vi "Measurement UI.vi"() -> ()   [LabVIEW 2021, in "channelGanging.lvlib"]
uses:
  channelGanging.lvlib
panel:
  in  "MeasGraphs":T1(tab)
  out "SourceCurrentGraph":waveform(dbl)[](graph) caption="AC"
  out "SourceVoltageGraph":waveform(dbl)[](graph) caption="AC"
  out "LoadCurrentGraph":waveform(dbl)[](graph) caption="AC"
  out "LoadVoltageGraph":waveform(dbl)[](graph) caption="AC"
  in  "Load channel mode":enum32{"Master", "Slave", "Slave- inverted"}[](array[ring])
  in  "Load resource names":string[](array[string])
  in  "Load input channels":i32[](array[numeric])
  in  "Source channel mode":enum32{"Master", "Slave", "Slave- inverted"}[](array[ring])
  in  "Source resource names":string[](array[string])
  in  "Source input channels":i32[](array[numeric])
  out "Load currents":dbl[](array[numeric])
  out "Load voltages":dbl[](array[numeric])
  out "Source currents":dbl[](array[numeric])
  out "Source voltages":dbl[](array[numeric])
  out "dt":dbl[](array[numeric])
  in  "MeasConfigurations":enum32{"Source Config", "Load Config"}(tab)
  in  "Source transient response":enum32{"Fast", "Normal", "Slow"}(ring) caption="TRANSIENT RESPONSE"
  in  "Source voltage level range":dbl=20.0 caption="VOLTAGE LEVEL RANGE" format="%#_6pV"
  in  "Source voltage level":dbl=2.0 caption="VOLTAGE LEVEL" format="%#_6pV"
  in  "Source channel parameters":T2(array[cluster]) caption="CHANNEL PARAMETERS"
  in  "Source current limit high":dbl=50.0 caption="CURRENT LIMIT HIGH" format="%#_6pA"
  in  "Source current limit range":dbl=40.0 caption="CURRENT LIMIT RANGE" format="%#_6pA"
  in  "Source limit symmetry":enum32{"Asymmetric", "Symmetric"}(ring) caption="LIMIT SYMMETRY"
  in  "Source current limit low":dbl=-0.6 caption="CURRENT  LIMIT LOW" format="%#_6pA"
  in  "Source system configuration":enum32{"Parallel", "Series"}(ring) caption="SYSTEM CONFIG"
  in  "Source sense":enum32{"Remote", "Local"}(ring) caption="SENSE"
  in  "Source aperture time":dbl=0.01 caption="APERTURE TIME" format="%.3ps"
  in  "Source compliance":string="Compliance"
  in  "Source timing":string="Timings"
  in  "Measurement time":dbl=1.0 caption="MEASUREMENT TIME" format="%.3ps"
  in  "Load transient response":enum32{"Fast", "Normal", "Slow"}(ring)=enum."Normal" caption="TRANSIENT RESPONSE"
  in  "Load timing":string="Timings"
  in  "Load compliance":string="Compliance"
  in  "Load aperture time":dbl=0.01 caption="APERTURE TIME" format="%.3ps"
  in  "Load Sense":enum32{"Remote", "Local"}(ring) caption="SENSE"
  in  "Load system configuration":enum32{"Parallel", "Series"}(ring) caption="SYSTEM CONFIG"
  in  "Load voltage limit low":dbl caption="VOLTAGE  LIMIT LOW" format="%#_6pV"
  in  "Load limit symmetry":enum32{"Asymmetric", "Symmetric"}(ring) caption="LIMIT SYMMETRY"
  in  "Load voltage limit range":dbl=6.0 caption="VOLTAGE LIMIT RANGE" format="%#_6pV"
  in  "Load voltage limit high":dbl=inf caption="VOLTAGE LIMIT HIGH" format="%#_6p"
  in  "Load current Level":dbl=30.0 caption="CURRENT LEVEL" format="%#_6pA"
  in  "Load current level range":dbl=50.0 caption="CURRENT LEVEL RANGE" format="%#_6pA"
  in  "Load channel parameters":T3(array[cluster]) caption="CHANNEL PARAMETERS"
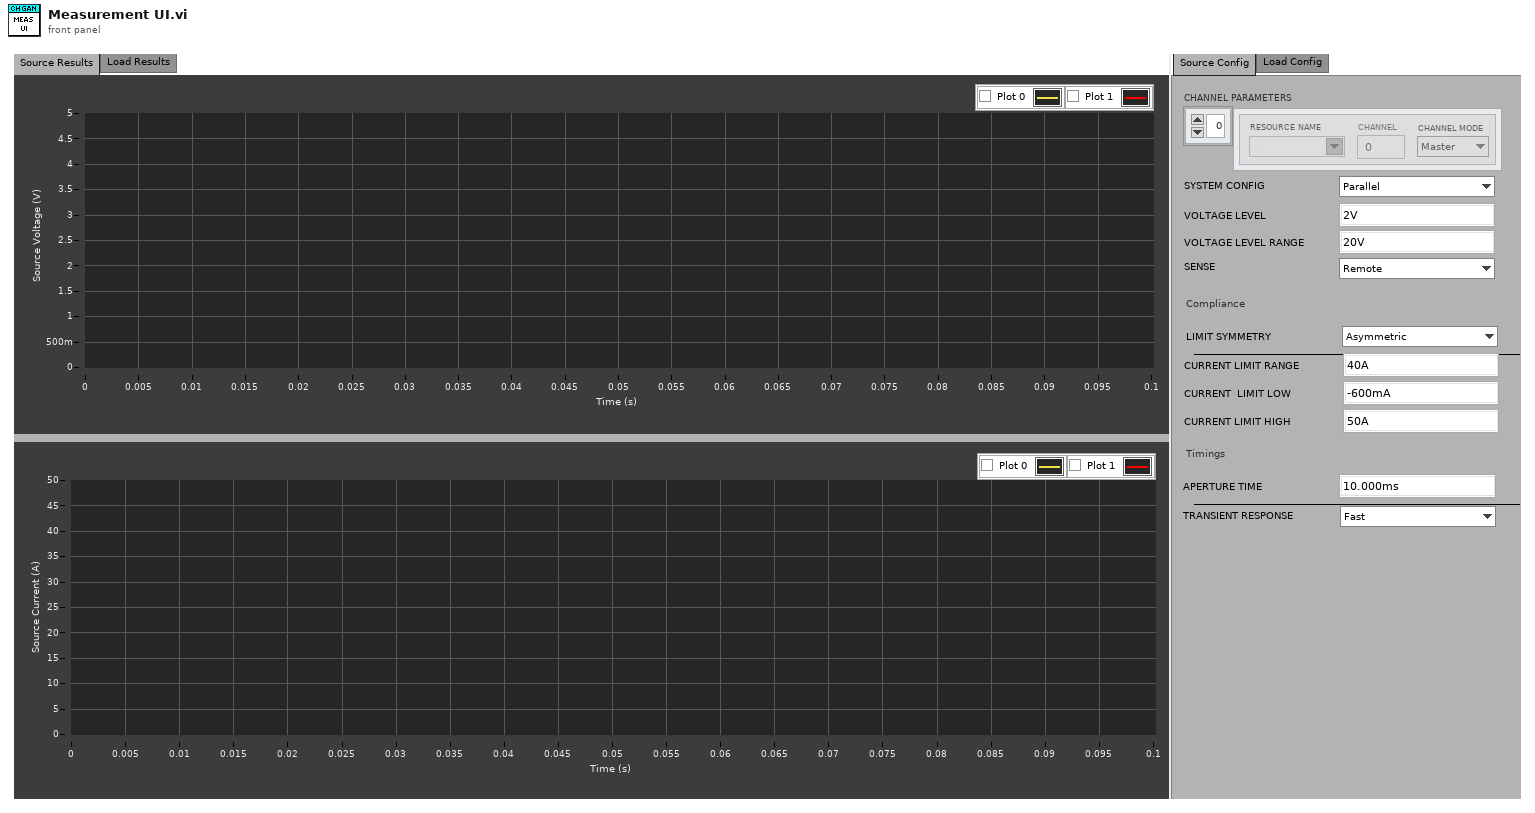
[diagram p1: front panel]
types:
  T1 = enum32{"Source Results", "Load Results", "Hidden Controls"}
  T2 = cluster{"PPSChannelMode":enum32{"Master", "Slave", "Slave- inverted"}, "PPSResourceName":refnum<k15>, "Input channel":i32}[]
  T3 = cluster{"EloadChannelMode":enum32{"Master", "Slave", "Slave- inverted"}, "EloadResourceName":refnum<k15>, "Load channel":i32}[]
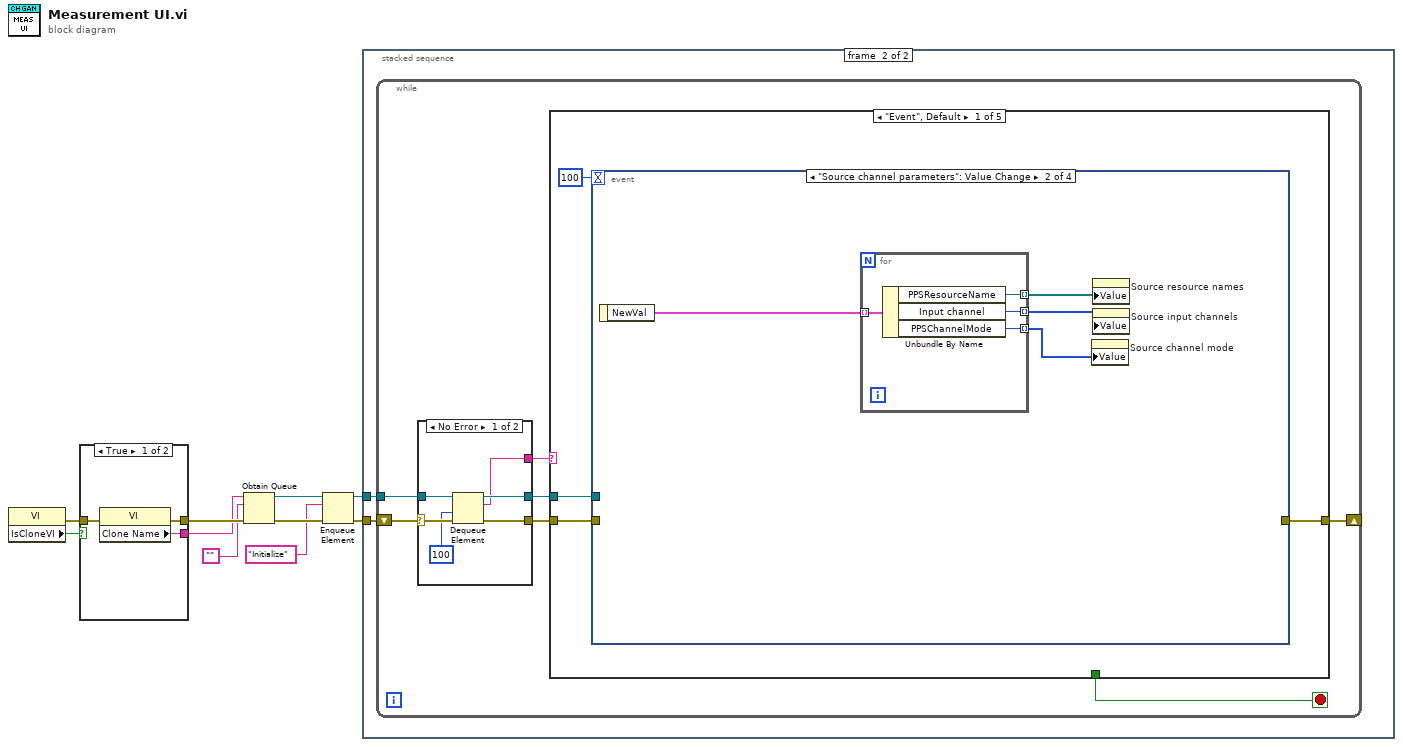
[diagram p0: block diagram]
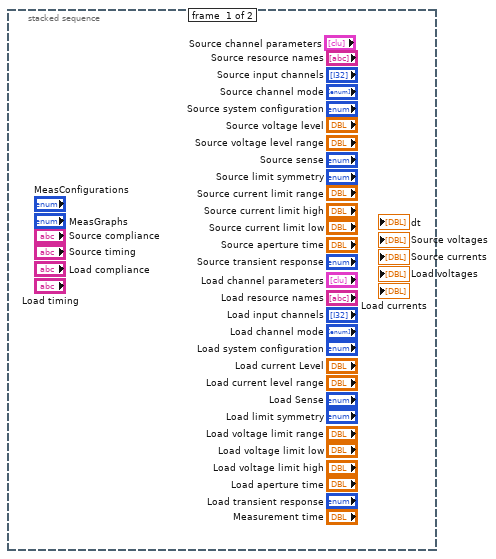
[diagram p2: hidden frame]
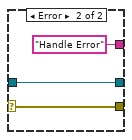
[diagram p3: hidden frame]
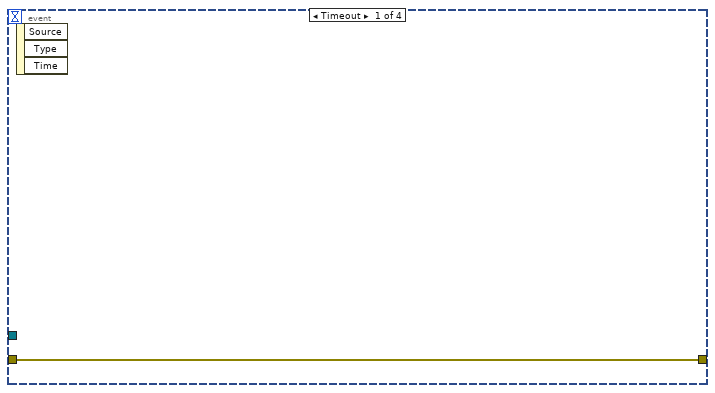
[diagram p4: hidden frame]
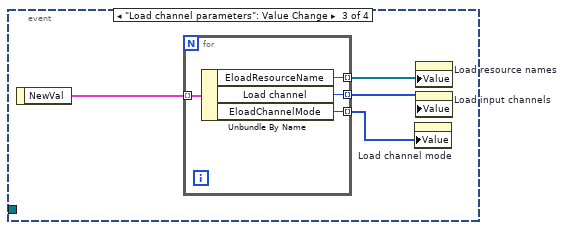
[diagram p5: hidden frame]
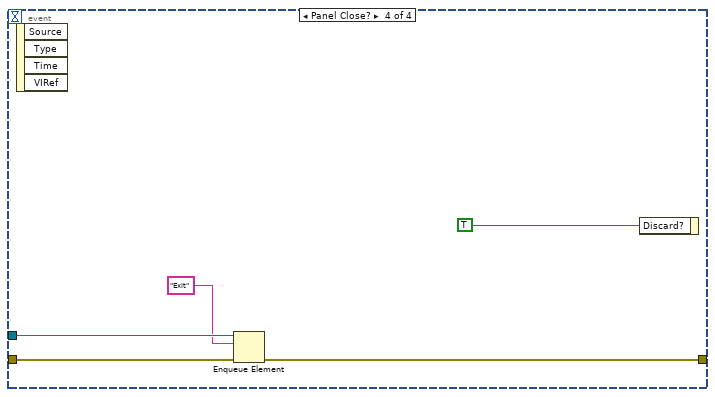
[diagram p6: hidden frame]
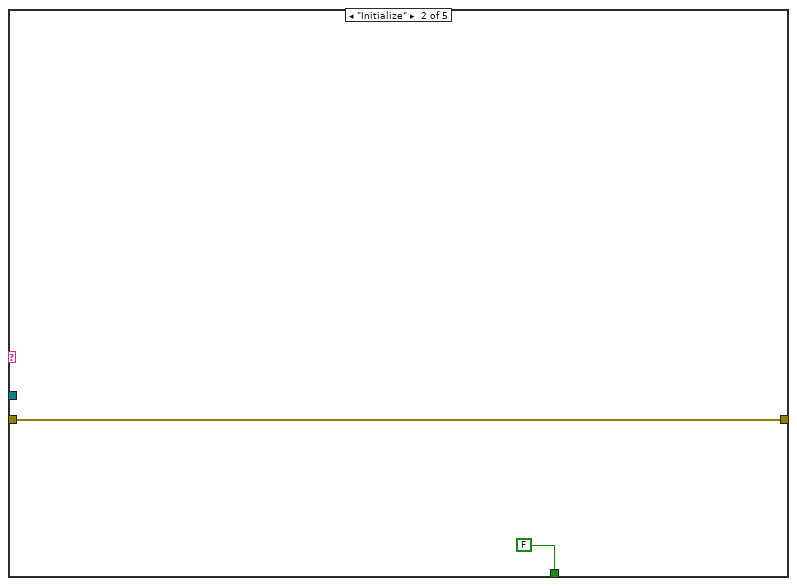
[diagram p7: hidden frame]
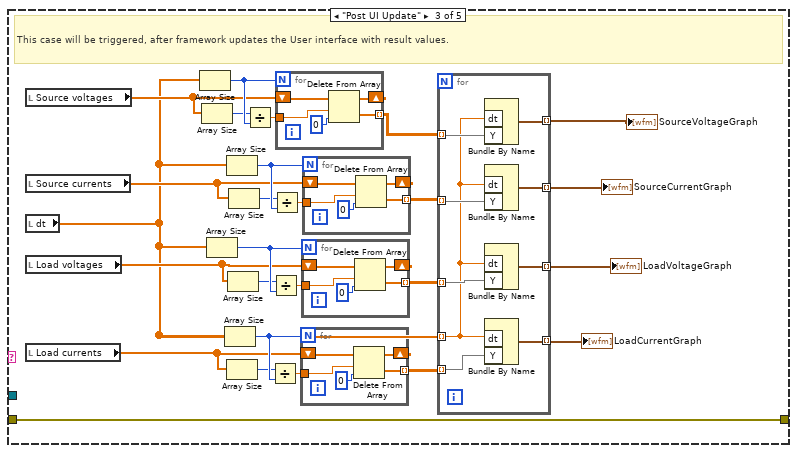
[diagram p8: hidden frame]
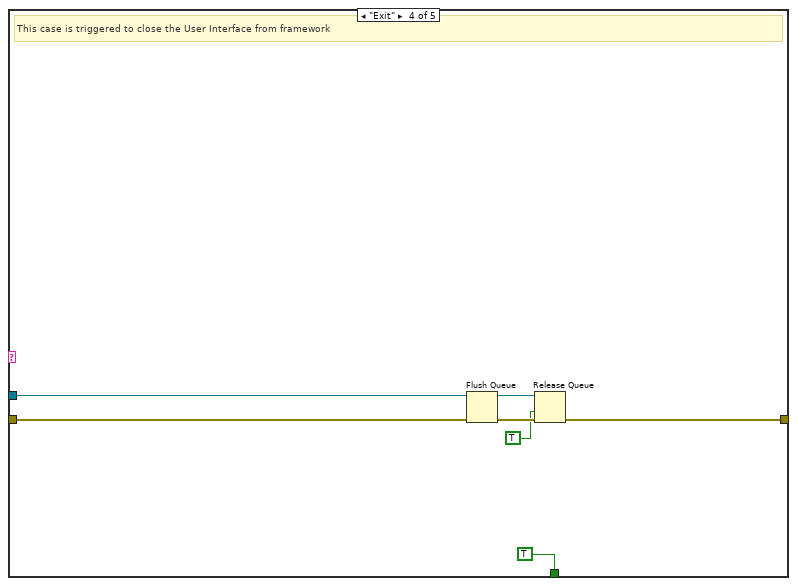
[diagram p9: hidden frame]
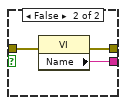
[diagram p11: hidden frame]
diagram:
  n1 = property class="VI"() -> (error out=w1:errorcluster, "IsCloneVI"=w2:bool)  [unwired: 2 in, 1 out]
  n2 = case shown="True" w2 {
    tunnel: [w13 w16] -> w10
    tunnel: [w12 w15] -> w9
    tunnel: w1 -> [w11 w14]
    frame True {
      n3 = property class="VI"(error in=w11) -> (error out=w13:errorcluster, "Clone Name"=w12:string)  [unwired: 1 in, 1 out]
    }
    frame False {
      n4 = property class="VI"(error in=w14) -> (error out=w16:errorcluster, "Name"=w15:string)  [unwired: 1 in, 1 out]
    }
  }
  n5 = Obtain Queue(name (unnamed)=w9, element data type="", error in (no error)=w10) -> (queue out=w6:refnum<queue>, error out=w8:errorcluster)  [unwired: 2 in, 1 out]
  n6 = Enqueue Element(queue=w6, element="Initialize", error in (no error)=w8) -> (queue out=w5:refnum<queue>, error out=w7:errorcluster)  [unwired: 1 in, 1 out]
  n7 = stacked-sequence {
    tunnel: w7 -> [_ w18]
    tunnel: w5 -> [_ w17]
    frame #0 {
    }
    frame #1 {
      n8 = while {
        shift-right: [w20] -> _
        shift-left: w18 -> [w25]
        tunnel: w17 -> [w23]
        stop <- w19 stop-if-true
        n9 = case shown="No Error" w25 {
          selector: w25 -> [w31 w34]
          tunnel: [w30 w34] -> w24
          tunnel: w23 -> [w29 w33]
          tunnel: [w28 w33] -> w22
          tunnel: [w27 "Handle Error"] -> w21
          frame No Error {
            n10 = Dequeue Element(queue=w29, timeout in ms (-1)=100, error in (no error)=w31) -> (queue out=w28:refnum<queue>, element=w27:string, error out=w30:errorcluster)  [unwired: 1 out]
          }
          frame Error {
          }
        }
        n11 = case shown="\"Event\", Default" w21 {
          tunnel: w24 -> [w37 w62 w88 w124 w125]
          tunnel: w22 -> [w35 _ _ w122 _]
          tunnel: [w38 w62 w88 w119 w125] -> w20
          tunnel: [_ FALSE _ TRUE _] -> w19
          frame "Event", Default {
            n12 = event shown="[1] \"Source channel parameters\": Value Change" {
              selector: _ -> [_ _ _ _]
              dyn-events: _ -> [_ _ _ _]
              timeout: 100 -> [_ _ _ _]
              tunnel: [w39 _ _ w58] -> w38
              tunnel: w37 -> [w39 _ _ w59]
              tunnel: w35 -> [_ _ _ w57]
              event Timeout {
                n13 = event-data() -> ()  [unwired: 1 in, 3 out]
              }
              event "Source channel parameters": Value Change {
                n14 = event-data() -> ("NewVal"=w43:T2)  [unwired: 1 in]
                n15 = for {
                  tunnel: w43 -> [w47] mode=indexing
                  tunnel: [w46] -> w42 mode=indexing
                  tunnel: [w45] -> w41 mode=indexing
                  tunnel: [w44] -> w40 mode=indexing
                  n16 = Unbundle By Name(w47) -> ("PPSResourceName"=w46:refnum<k15>, "Input channel"=w45:i32, "PPSChannelMode"=w44:enum32{"Master", "Slave", "Slave- inverted"})
                }
                n17 = property on="Source channel mode" class="Arr (strict)"("Value"=w40) -> ()  [unwired: 2 in, 2 out]
                n18 = property on="Source resource names" class="Arr (strict)"("Value"=w42) -> ()  [unwired: 2 in, 2 out]
                n19 = property on="Source input channels" class="Arr (strict)"("Value"=w41) -> ()  [unwired: 2 in, 2 out]
              }
              event "Load channel parameters": Value Change {
                n20 = event-data() -> ("NewVal"=w48:T3)  [unwired: 1 in]
                n21 = for {
                  tunnel: w48 -> [w55] mode=indexing
                  tunnel: [w54] -> w49 mode=indexing
                  tunnel: [w53] -> w50 mode=indexing
                  tunnel: [w52] -> w51 mode=indexing
                  n22 = Unbundle By Name(w55) -> ("EloadResourceName"=w54:refnum<k15>, "Load channel"=w53:i32, "EloadChannelMode"=w52:enum32{"Master", "Slave", "Slave- inverted"})
                }
                n23 = property on="Load channel mode" class="Arr (strict)"("Value"=w51) -> ()  [unwired: 2 in, 2 out]
                n24 = property on="Load resource names" class="Arr (strict)"("Value"=w49) -> ()  [unwired: 2 in, 2 out]
                n25 = property on="Load input channels" class="Arr (strict)"("Value"=w50) -> ()  [unwired: 2 in, 2 out]
              }
              event Panel Close? {
                n26 = event-data() -> ()  [unwired: 1 in, 4 out]
                n27 = Enqueue Element(queue=w57, element="Exit", error in (no error)=w59) -> (error out=w58:errorcluster)  [unwired: 1 in, 2 out]
                n28 = event-data("Discard?"=TRUE) -> ()  [unwired: 1 in, 1 out]
              }
            }
          }
          frame "Initialize" {
          }
          frame "Post UI Update" {
            # "This case will be triggered, after framework updates the User interface with result values."
            n29 = local read "Source voltages"() -> (w65:dbl[])
            n30 = local read "Source currents"() -> (w66:dbl[])
            n31 = local read "dt"() -> (w63:dbl[])
            n32 = local read "Load voltages"() -> (w64:dbl[])
            n33 = local read "Load currents"() -> (w84:dbl[])
            n34 = Array Size(array=w63) -> (size(s)=w78:i32)
            n35 = Array Size(array=w65) -> (size(s)=w76:i32)
            n36 = Array Size(array=w63) -> (size(s)=w81:i32)
            n37 = Array Size(array=w63) -> (size(s)=w87:i32)
            n38 = Array Size(array=w63) -> (size(s)=w75:i32)
            n39 = Array Size(array=w84) -> (size(s)=w85:i32)
            n40 = Array Size(array=w64) -> (size(s)=w79:i32)
            n41 = Array Size(array=w66) -> (size(s)=w73:i32)
            n42 = Divide(x=w76, y=w78) -> (x/y=w77:dbl)
            n43 = Divide(x=w85, y=w87) -> (x/y=w86:dbl)
            n44 = Divide(x=w79, y=w81) -> (x/y=w80:dbl)
            n45 = Divide(x=w73, y=w75) -> (x/y=w74:dbl)
            n46 = for {
              N: w78 -> [_]
              tunnel: w77 -> [w95]
              tunnel: [w96] -> w71 mode=indexing
              shift-right: [w97] -> _
              shift-left: w65 -> [w98]
              n47 = Delete From Array(array=w98, length=w95, index=0) -> (deleted portion=w96:dbl[], array with subset deleted=w97:dbl[])
            }
            n48 = for {
              N: w87 -> [_]
              tunnel: w86 -> [w114]
              tunnel: [w115] -> w83 mode=indexing
              shift-right: [w116] -> _
              shift-left: w84 -> [w117]
              n49 = Delete From Array(array=w117, length=w114, index=0) -> (deleted portion=w115:dbl[], array with subset deleted=w116:dbl[])
            }
            n50 = for {
              N: w81 -> [_]
              tunnel: w80 -> [w100]
              tunnel: [w101] -> w72 mode=indexing
              shift-right: [w102] -> _
              shift-left: w64 -> [w103]
              n51 = Delete From Array(array=w103, length=w100, index=0) -> (deleted portion=w101:dbl[], array with subset deleted=w102:dbl[])
            }
            n52 = for {
              N: w75 -> [_]
              tunnel: w74 -> [w90]
              tunnel: [w91] -> w70 mode=indexing
              shift-right: [w92] -> _
              shift-left: w66 -> [w93]
              n53 = Delete From Array(array=w93, length=w90, index=0) -> (deleted portion=w91:dbl[], array with subset deleted=w92:dbl[])
            }
            n54 = for {
              tunnel: w63 -> [w104] mode=indexing
              tunnel: w83 -> [w112] mode=indexing
              tunnel: [w111] -> w82 mode=indexing
              tunnel: w72 -> [w110] mode=indexing
              tunnel: w71 -> [w109] mode=indexing
              tunnel: w70 -> [w108] mode=indexing
              tunnel: [w107] -> w69 mode=indexing
              tunnel: [w106] -> w68 mode=indexing
              tunnel: [w105] -> w67 mode=indexing
              n55 = Bundle By Name("dt"=w104, "Y"=w109) -> (w106:waveform(dbl))  [unwired: 1 in]
              n56 = Bundle By Name("dt"=w104, "Y"=w108) -> (w107:waveform(dbl))  [unwired: 1 in]
              n57 = Bundle By Name("dt"=w104, "Y"=w110) -> (w105:waveform(dbl))  [unwired: 1 in]
              n58 = Bundle By Name("dt"=w104, "Y"=w112) -> (w111:waveform(dbl))  [unwired: 1 in]
            }
            "SourceVoltageGraph" <- w68
            "SourceCurrentGraph" <- w69
            "LoadVoltageGraph" <- w67
            "LoadCurrentGraph" <- w82
          }
          frame "Exit" {
            # "This case is triggered to close the User Interface from framework"
            n59 = Flush Queue(queue=w122, error in (no error)=w124) -> (queue out=w121:refnum<queue>, error out=w120:errorcluster)  [unwired: 1 out]
            n60 = Release Queue(queue=w121, force destroy? (F)=TRUE, error in (no error)=w120) -> (error out=w119:errorcluster)  [unwired: 2 out]
          }
          frame "Handle Error" {
          }
        }
      }
    }
  }
